vi "test compare I32.vi"(8 "error in (no error)":errorcluster, 11 "Passing test in":refnum<class "LUnit Test 3.lvclass">) -> (0 "error out":errorcluster, 3 "Passing test out":refnum<class "LUnit Test 3.lvclass">)   [LabVIEW 2020, in "LUnit Test 3.lvclass"]
uses:
  LUnit Test 3.lvclass
  <vilib>/Astemes/LUnit/Test Case.lvclass/Test Case.ctl
  <vilib>/Astemes/LUnit/Palette/Pass If Equal.vi/cbf50e99-f124-4847-863a-8e9794d3dede.vi
  <vilib>/Astemes/LUnit/Core/LUnit Test Case/Private/Append Pass Result.vi
  <vilib>/Astemes/LUnit/Core/LUnit Test Case/Private/Append Fail Result.vi
  <vilib>/Astemes/LUnit/Palette/Pass If Equal.vi/cbf50e99-f124-4847-863a-8e9794d3dede.vi/9c5d11cd-9439-4240-a1ee-d9baace9c924.vi
  <vilib>/Astemes/LUnit/Core/LUnit Test Case/Private/Run In UI.vi
  <vilib>/Utility/error.llb/Clear Errors.vi
  LUnit Test 3.lvclass/LUnit Test 3.ctl
  ec809e2e-37fd-424c-a52d-1cfb1da04956.vi
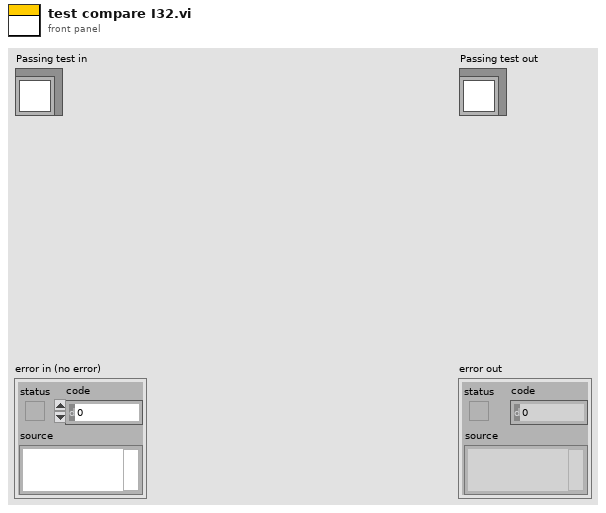
[diagram p1: front panel]
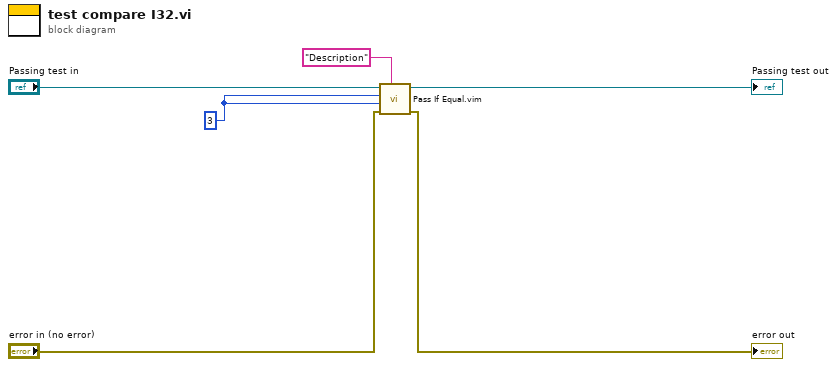
[diagram p0: block diagram]
diagram:
  w2 = 3
  n1 = call "Pass If Equal.vim"("Description"="Description", "error in (no error)"="error in (no error)", "Actual"=w2, "Expected"=w2, "LUnit Test Case In"="Passing test in") -> ("error out"=→"error out":errorcluster, "LUnit Test Case Out"=→"Passing test out":refnum<class "LUnit Test 3.lvclass">)  [unwired: 5 in]
